vi "Set SimulationFlag.vi"(8 "error in (no error)":errorcluster, 9 "Unit ID":u16, 10 "Simulation?":bool, 11 "Device in":refnum<class "DAQ_Device.lvclass">) -> (0 "error out":errorcluster, 3 "Device out":refnum<class "DAQ_Device.lvclass">)   [LabVIEW 2023, in "DAQ_Device.lvclass"]
uses:
  DAQ_Device.lvclass
  DAQ_Device.lvclass/DAQ_Device.ctl
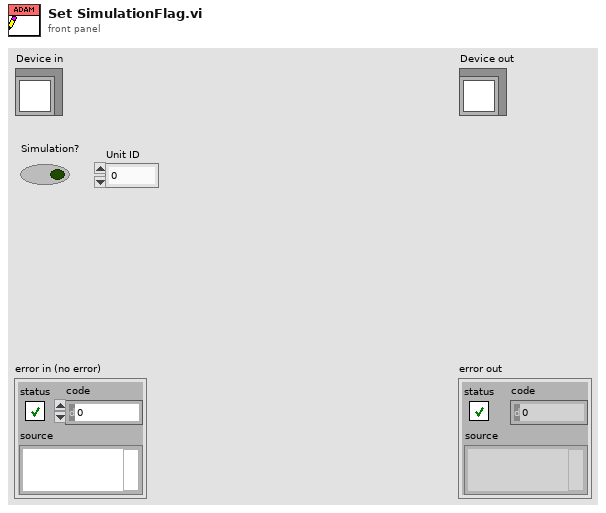
[diagram p1: front panel]
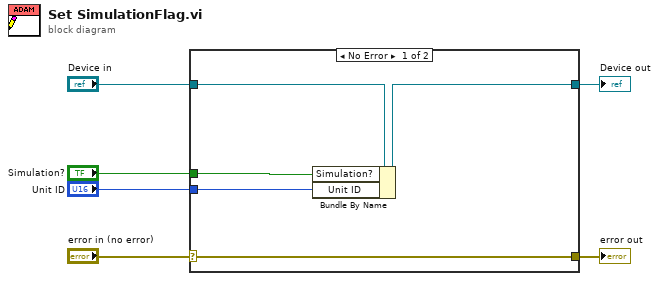
[diagram p0: block diagram]
diagram:
  n1 = case shown="No Error" "error in (no error)" {
    selector: "error in (no error)" -> [w11 w12]
    tunnel: [w11 w12] -> w5
    tunnel: [w9 w13] -> w3
    tunnel: "Device in" -> [w10 w13]
    tunnel: "Simulation?" -> [w8 _]
    tunnel: "Unit ID" -> [w7 _]
    frame No Error {
      n2 = Bundle By Name(cluster=w10, "Simulation?"=w8, "Unit ID"=w7) -> (w9:refnum<class "DAQ_Device.lvclass">)
    }
    frame Error {
    }
  }
  "error out" <- w5
  "Device out" <- w3
